vi "Initial Pie Chart.vi"(10 "中心位置":T2={"Cent X"=273.0, "Cent Y"=190.0, "R"=180.0, "Color1Number"=20.0, "Color2Number"=50.0, "Color3Number"=40.0, "Color4Number"=70.0, "Color5Number"=90.0}, 11 "Pie Image In":T3(plugin-control)) -> (2 "Precent Output":T1, 3 "Pie Image Out":T3(plugin-control))   [LabVIEW 2015]
panel:
  out "XY输出":cluster{"X":dbl, "Y":dbl}
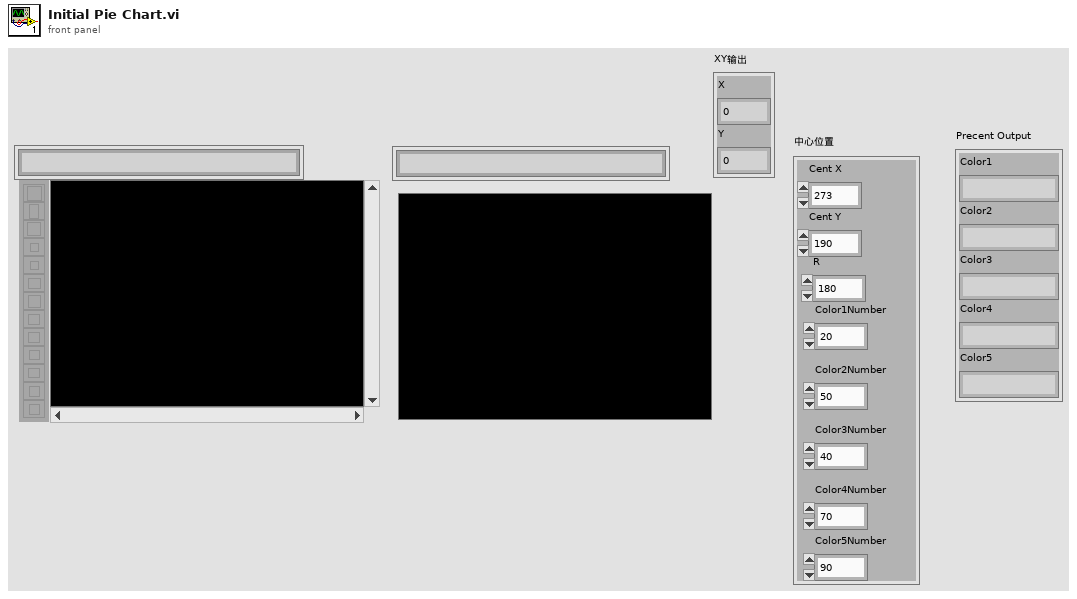
[diagram p1: front panel]
types:
  T1 = cluster{"Color1":string, "Color2":string, "Color3":string, "Color4":string, "Color5":string}
  T2 = cluster{"Cent X":dbl, "Cent Y":dbl, "R":dbl, "Color1Number":dbl, "Color2Number":dbl, "Color3Number":dbl, "Color4Number":dbl, "Color5Number":dbl}
  T3 = typedef "IMAQ Image.ctl" = refnum<image>
  T4 = cluster{"Left":i32, "Top":i32, "Right":i32, "Bottom":i32}
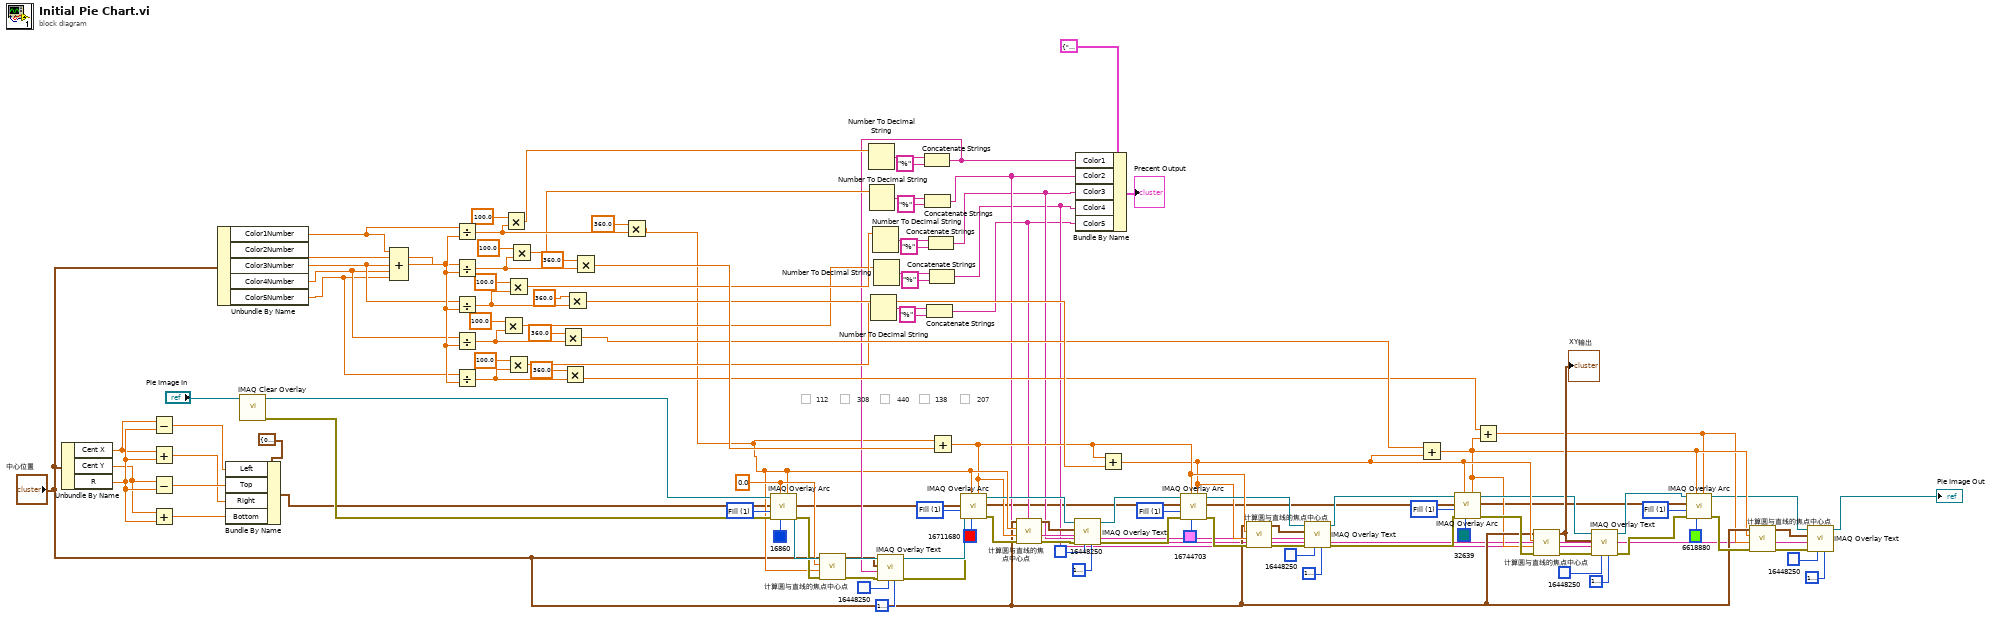
[diagram p0: block diagram]
diagram:
  w68 = u32 1 items=["Frame", "Fill"] ("Drawing Mode (Frame)")
  w71 = u32 1 items=["Frame", "Fill"] ("Drawing Mode (Frame)")
  w73 = u32 1 items=["Frame", "Fill"] ("Drawing Mode (Frame)")
  w74 = u32 1 items=["Frame", "Fill"] ("Drawing Mode (Frame)")
  w109 = u32 1 items=["Frame", "Fill"] ("Drawing Mode (Frame)")
  w46 = 0.0 ("Start Angle (degrees)")
  # "207"
  # "308"
  # "440"
  # "138"
  # "112"
  n1 = Unbundle By Name("中心位置") -> ("Cent X"=w106:dbl, "Cent Y"=w107:dbl, "R"=w110:dbl)
  n2 = Subtract(x=w106, y=w110) -> (x-y=w114:dbl)
  n3 = Add(x=w106, y=w110) -> (x+y=w112:dbl)
  n4 = Subtract(x=w107, y=w110) -> (x-y=w113:dbl)
  n5 = Add(x=w107, y=w110) -> (x+y=w111:dbl)
  n6 = Unbundle By Name("中心位置") -> ("Color1Number"=w102:dbl, "Color2Number"=w100:dbl, "Color3Number"=w99:dbl, "Color4Number"=w98:dbl, "Color5Number"=w97:dbl)
  n7 = Bundle By Name(cluster=T4 {"Left"=0, "Top"=0, "Right"=0, "Bottom"=0} ("Bounding Rectangle"), "Left"=w114, "Top"=w113, "Right"=w112, "Bottom"=w111) -> (w2:T4)
  n8 = call "IMAQ Clear Overlay"("Image"="Pie Image In") -> ("error out"=w104:errorcluster, "Image Out"=w103:T3)  [unwired: 9 in]
  n9 = Compound Arithmetic op=ADD(w102, w100, w99, w98, w97) -> (w101:dbl)
  n10 = Divide(x=w102, y=w101) -> (x/y=w67:dbl)
  n11 = Divide(x=w100, y=w101) -> (x/y=w63:dbl)
  n12 = Divide(x=w99, y=w101) -> (x/y=w60:dbl)
  n13 = Divide(x=w98, y=w101) -> (x/y=w57:dbl)
  n14 = Divide(x=w97, y=w101) -> (x/y=w54:dbl)
  n15 = Multiply(x=100.0, y=w57) -> (x*y=w56:dbl)
  n16 = Multiply(x=100.0, y=w67) -> (x*y=w65:dbl)
  n17 = Multiply(x=100.0, y=w60) -> (x*y=w59:dbl)
  n18 = Multiply(x=100.0, y=w54) -> (x*y=w53:dbl)
  n19 = Multiply(x=100.0, y=w63) -> (x*y=w62:dbl)
  n20 = Multiply(x=360.0, y=w57) -> (x*y=w78:dbl)
  n21 = Multiply(x=360.0, y=w54) -> (x*y=w76:dbl)
  n22 = Multiply(x=360.0, y=w60) -> (x*y=w80:dbl)
  n23 = Multiply(x=360.0, y=w63) -> (x*y=w82:dbl)
  n24 = Multiply(x=360.0, y=w67) -> (x*y=w39:dbl)
  n25 = call "IMAQ Overlay Arc"("End Angle (degrees)"=w39, "Color"=u32 16860, "Start Angle (degrees)"=w46, "error in (no error)"=w104, "Drawing Mode (Frame)"=w109, "Bounding Rectangle"=w2, "Image"=w103) -> ("error out"=w45:errorcluster, "Image Out"=w52:T3)  [unwired: 3 in]
  n26 = call "计算圆与直线的焦点中心点.vi"("error in (no error)"=w45, "结束角度"=w39, "起始角度"=w46, "中心位置"="中心位置") -> ("error out"=w44:errorcluster, "XY输出"=w1:cluster{"X":dbl, "Y":dbl})  [unwired: 6 in]
  n27 = Number To Decimal String(number=w65) -> (decimal integer string=w94:string)  [unwired: 1 in]
  n28 = Number To Decimal String(number=w62) -> (decimal integer string=w93:string)  [unwired: 1 in]
  n29 = Number To Decimal String(number=w53) -> (decimal integer string=w86:string)  [unwired: 1 in]
  n30 = Number To Decimal String(number=w59) -> (decimal integer string=w90:string)  [unwired: 1 in]
  n31 = Number To Decimal String(number=w56) -> (decimal integer string=w89:string)  [unwired: 1 in]
  n32 = Concatenate Strings(w94, "%" ("字符串")) -> (w49:string)
  n33 = call "IMAQ Overlay Text"("BG Color (Transparent)"=u32 16777216, "Text Color (black)"=u32 16448250, "error in (no error)"=w44, "String"=w49, "Origin"=w1, "Image"=w52) -> ("error out"=w50:errorcluster, "Image Out"=w51:T3)  [unwired: 4 in]
  n34 = Concatenate Strings(w93, "%" ("字符串")) -> (w6:string)
  n35 = Concatenate Strings(w86, "%" ("字符串")) -> (w3:string)
  n36 = Concatenate Strings(w90, "%" ("字符串")) -> (w5:string)
  n37 = Concatenate Strings(w89, "%" ("字符串")) -> (w4:string)
  n38 = Add(x=w39, y=w82) -> (x+y=w28:dbl)
  n39 = call "IMAQ Overlay Arc"("End Angle (degrees)"=w28, "Color"=u32 16711680, "Start Angle (degrees)"=w39, "error in (no error)"=w50, "Drawing Mode (Frame)"=w74, "Bounding Rectangle"=w2, "Image"=w51) -> ("error out"=w40:errorcluster, "Image Out"=w37:T3)  [unwired: 3 in]
  n40 = call "计算圆与直线的焦点中心点.vi"("error in (no error)"=w40, "结束角度"=w28, "起始角度"=w39, "中心位置"="中心位置") -> ("error out"=w43:errorcluster, "XY输出"=w38:cluster{"X":dbl, "Y":dbl})  [unwired: 6 in]
  n41 = call "IMAQ Overlay Text"("BG Color (Transparent)"=u32 16777216, "Text Color (black)"=u32 16448250, "error in (no error)"=w43, "String"=w6, "Origin"=w38, "Image"=w37) -> ("error out"=w35:errorcluster, "Image Out"=w36:T3)  [unwired: 4 in]
  n42 = Bundle By Name(cluster=T1 {"Color1"="", "Color2"="", "Color3"="", "Color4"="", "Color5"=""}, "Color1"=w49, "Color2"=w6, "Color3"=w5, "Color4"=w4, "Color5"=w3) -> (→"Precent Output":T1)
  n43 = Add(x=w28, y=w80) -> (x+y=w20:dbl)
  n44 = call "IMAQ Overlay Arc"("End Angle (degrees)"=w20, "Color"=u32 16744703, "Start Angle (degrees)"=w28, "error in (no error)"=w35, "Drawing Mode (Frame)"=w73, "Bounding Rectangle"=w2, "Image"=w36) -> ("error out"=w30:errorcluster, "Image Out"=w27:T3)  [unwired: 3 in]
  n45 = call "计算圆与直线的焦点中心点.vi"("error in (no error)"=w30, "结束角度"=w20, "起始角度"=w28, "中心位置"="中心位置") -> ("error out"=w31:errorcluster, "XY输出"=w34:cluster{"X":dbl, "Y":dbl})  [unwired: 6 in]
  n46 = call "IMAQ Overlay Text"("BG Color (Transparent)"=u32 16777216, "Text Color (black)"=u32 16448250, "error in (no error)"=w31, "String"=w5, "Origin"=w34, "Image"=w27) -> ("error out"=w29:errorcluster, "Image Out"=w26:T3)  [unwired: 4 in]
  n47 = Add(x=w78, y=w20) -> (x+y=w11:dbl)
  n48 = call "IMAQ Overlay Arc"("End Angle (degrees)"=w11, "Color"=u32 32639, "Start Angle (degrees)"=w20, "error in (no error)"=w29, "Drawing Mode (Frame)"=w68, "Bounding Rectangle"=w2, "Image"=w26) -> ("error out"=w21:errorcluster, "Image Out"=w19:T3)  [unwired: 3 in]
  n49 = Add(x=w76, y=w11) -> (x+y=w10:dbl)
  n50 = call "计算圆与直线的焦点中心点.vi"("error in (no error)"=w21, "结束角度"=w11, "起始角度"=w20, "中心位置"="中心位置") -> ("error out"=w25:errorcluster, "XY输出"=w22:cluster{"X":dbl, "Y":dbl})  [unwired: 6 in]
  "XY输出" <- w22
  n51 = call "IMAQ Overlay Text"("BG Color (Transparent)"=u32 16777216, "Text Color (black)"=u32 16448250, "error in (no error)"=w25, "String"=w4, "Origin"=w22, "Image"=w19) -> ("error out"=w14:errorcluster, "Image Out"=w18:T3)  [unwired: 4 in]
  n52 = call "IMAQ Overlay Arc"("End Angle (degrees)"=w10, "Color"=u32 6618880, "Start Angle (degrees)"=w11, "error in (no error)"=w14, "Drawing Mode (Frame)"=w71, "Bounding Rectangle"=w2, "Image"=w18) -> ("error out"=w13:errorcluster, "Image Out"=w8:T3)  [unwired: 3 in]
  n53 = call "计算圆与直线的焦点中心点.vi"("error in (no error)"=w13, "结束角度"=w10, "起始角度"=w11, "中心位置"="中心位置") -> ("error out"=w15:errorcluster, "XY输出"=w9:cluster{"X":dbl, "Y":dbl})  [unwired: 6 in]
  n54 = call "IMAQ Overlay Text"("BG Color (Transparent)"=u32 16777216, "Text Color (black)"=u32 16448250, "error in (no error)"=w15, "String"=w3, "Origin"=w9, "Image"=w8) -> ("Image Out"=→"Pie Image Out":T3)  [unwired: 4 in, 1 out]
